vi "Sleep.vi"(8 "error in (no error)":errorcluster, 11 "CellPhone ISleepable in":refnum<class "ISleepableCellPhone.lvclass">) -> (0 "error out":errorcluster, 3 "CellPhone ISleepable out":refnum<class "ISleepableCellPhone.lvclass">)   [LabVIEW 2009, in "ISleepableCellPhone.lvclass"]
uses:
  ISleepableCellPhone.lvclass
  CellPhone.lvclass
  Source/IUnknown Class/IUnknown.lvclass
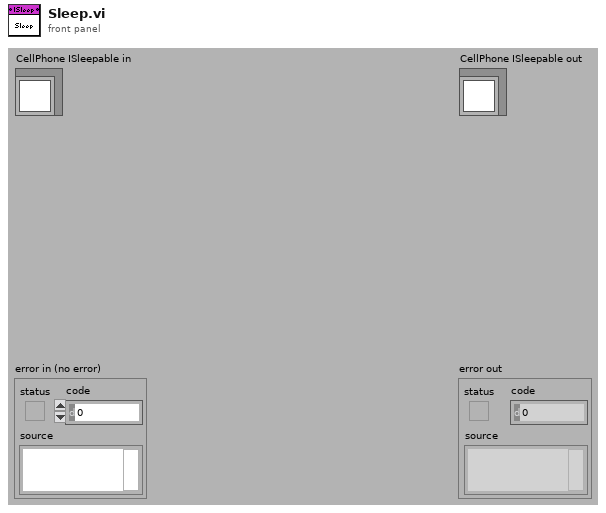
[diagram p1: front panel]
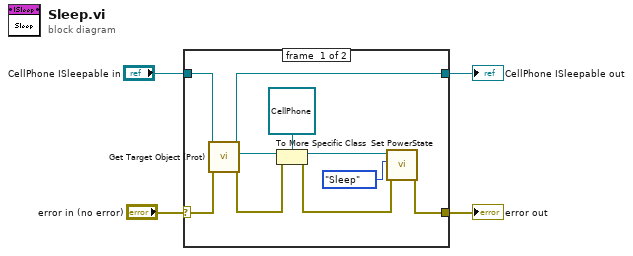
[diagram p0: block diagram]
diagram:
  n1 = case shown="No Error" "error in (no error)" {
    selector: "error in (no error)" -> [w5 w15]
    tunnel: "CellPhone ISleepable in" -> [w14 w16]
    tunnel: [w13 w16] -> w3
    tunnel: [w7 w15] -> w2
    frame #0 {
      n2 = call "Get Target Object (Prot).vi"("error in (no error)"=w5, "IUnknown in"=w14) -> ("error out"=w9:errorcluster, "Target Object"=w10:refnum<class "Interfaceable.lvclass">, "IUnknown out"=w13:refnum<class "ISleepableCellPhone.lvclass">)  [unwired: 7 in]
      n3 = To More Specific Class(target class=refnum<class "CellPhone.lvclass"> refnum ("CellPhone"), reference=w10, error in=w9) -> (specific class reference=w11:refnum<class "CellPhone.lvclass">, error out=w8:errorcluster)
      n4 = call "Set PowerState.vi"("error in (no error)"=w8, "PowerState"=enum16{"Off", "Sleep", "On"}."Sleep", "CellPhone in"=w11) -> ("error out"=w7:errorcluster)  [unwired: 7 in, 1 out]
    }
    frame #1 {
    }
  }
  "error out" <- w2
  "CellPhone ISleepable out" <- w3
